vi "Rx Core 2945 2955.vi"(0 "rx.ddc parameters":T1[](array[typedef]) {"frequency shift" format="%#.48g"}, 1 "rx.samples to acquire":u32, 2 "Simulate Data":bool, 3 "rx.abort":bool, 4 "rx.stream enable":bool[](array[boolean]), 5 "rx.start trigger":bool, 6 "rx.reset":bool=TRUE, 7 "fifo 2":refnum<k21>, 10 "fifo 0":refnum<k21>, 11 "fifo 3":refnum<k21>, 12 "fifo 1":refnum<k21>) -> (13 "rx.dsp reset done":bool, 14 "rx.state":T3, 15 "rx.samples processed":u32, 17 "rx.number of fifo overflows":u32, 18 "rx.number of iq data overflows":u64[](array[numeric]))   [LabVIEW 2016]
uses:
  Stream Control State.ctl
  DDC Parameters.ctl
  <instrlib>/_niInstr/DSP/v1/Shared/Public/IQ Impairments.ctl
  <vilib>/rvi/eio/common/nirviEmuTemplateMethod_errors.vi
  <instrlib>/_niInstr/DSP/v1/FPGA/Public/Sub VIs/Data Conversion/I16 to IQ - 1 spc - S18.1.vi
  <instrlib>/_niInstr/Basic Elements/v1/FPGA/Private/Count Up U32.vi
  <vilib>/eio/EIONode/EIONode.xnode
  <instrlib>/_niInstr/Basic Elements/v1/FPGA/niInstr Basic Elements v1 FPGA.lvlib
  <instrlib>/_niInstr/DSP/v1/FPGA/niInstr DSP v1 FPGA.lvlib
  <instrlib>/_niInstr/DSP/v1/Shared/niInstr DSP v1 Shared.lvlib
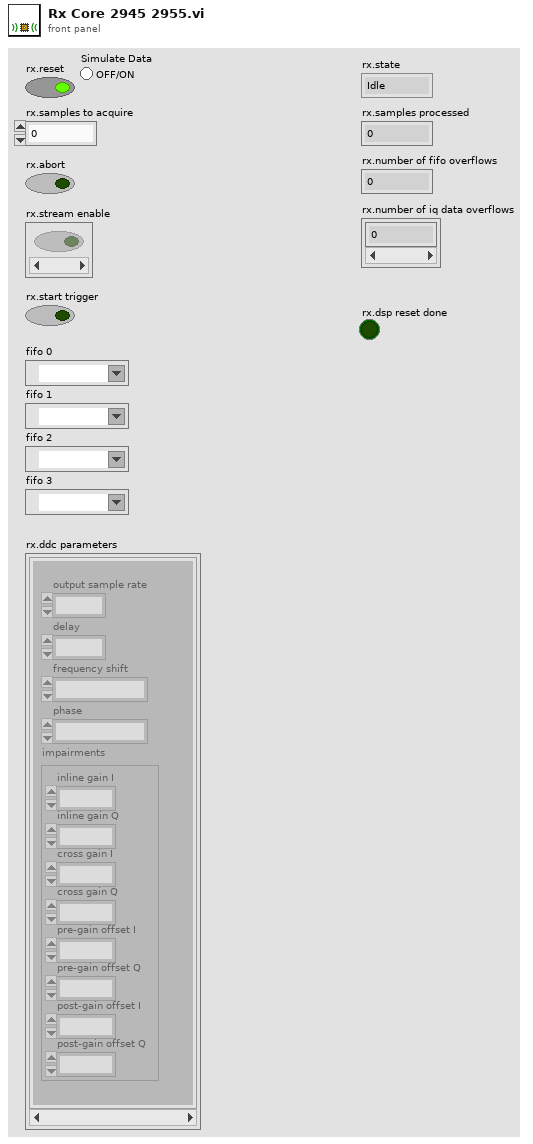
[diagram p1: front panel]
types:
  T1 = typedef "DDC Parameters.ctl" = cluster{"output sample rate":fxp<+,48,1>, "delay":fxp<+/-,16,0>, "frequency shift":fxp<+/-,48,0>, "impairments":T2, "phase":fxp<+/-,21,0>}
  T2 = typedef "niInstr DSP v1 Shared.lvlib/IQ Impairments.ctl" = cluster{"inline gain I":fxp<+/-,18,1>, "inline gain Q":fxp<+/-,18,1>, "cross gain I":fxp<+/-,18,1>, "cross gain Q":fxp<+/-,18,1>, "pre-gain offset I":fxp<+/-,18,1>, "pre-gain offset Q":fxp<+/-,18,1>, "post-gain offset I":fxp<+/-,18,1>, "post-gain offset Q":fxp<+/-,18,1>}
  T3 = typedef "Stream Control State.ctl" = enum16{"Idle", "Active"}
  T4 = typedef "niInstr DSP v1 Shared.lvlib/IQ Data.ctl" = cluster{"I":fxp<+/-,18,1>, "Q":fxp<+/-,18,1>, "overflow":bool}
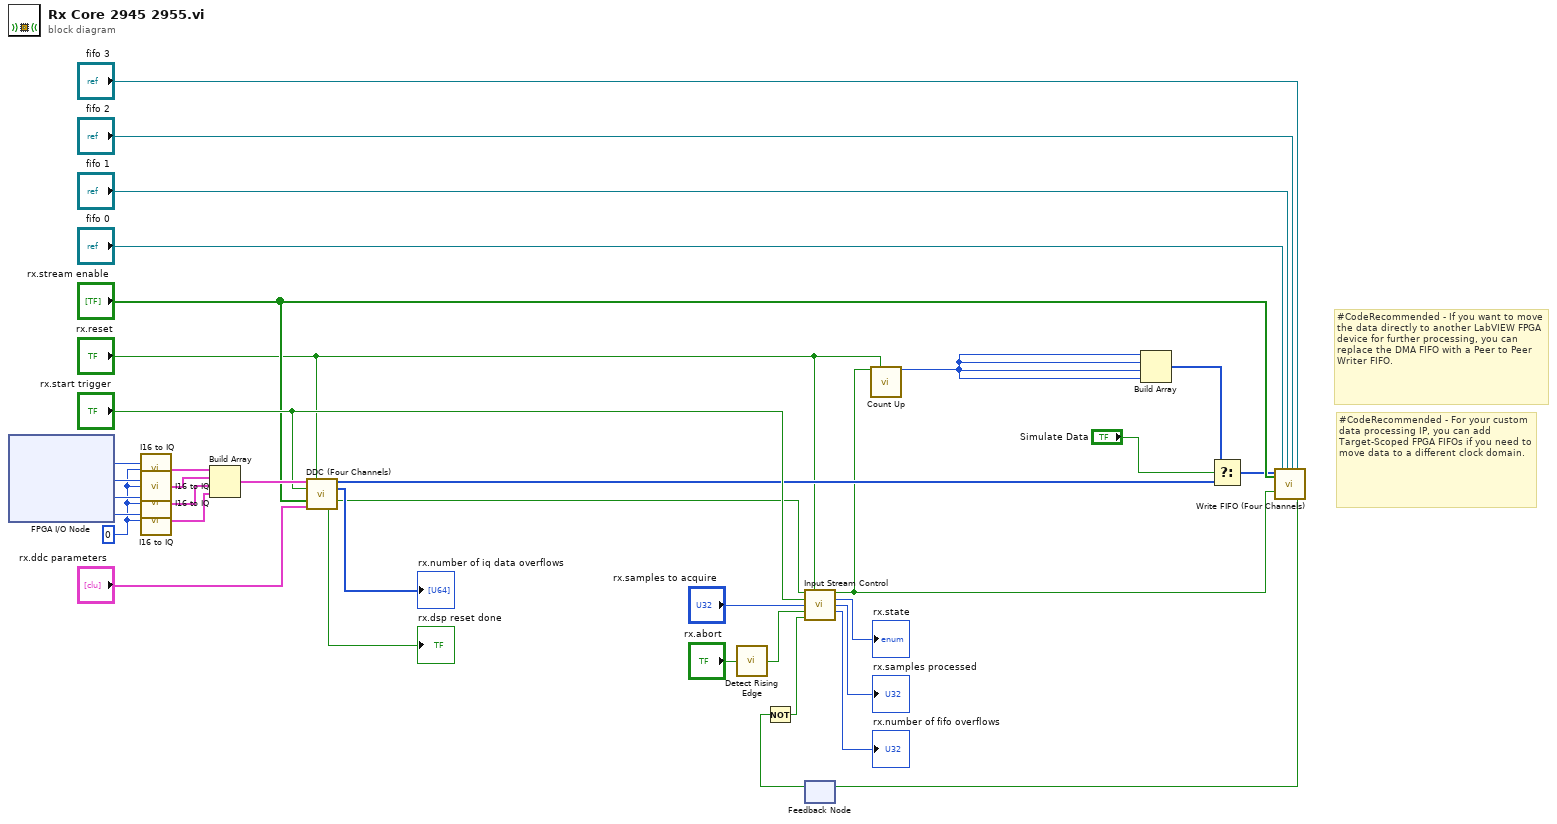
[diagram p0: block diagram]
diagram:
  w22 = i16 0 ("Q")
  # "#CodeRecommended - For your custom data processing IP, you can add Target-Scoped FPGA FIFOs if you need to move data to a different clock domain."
  # "#CodeRecommended - If you want to move the data directly to another LabVIEW FPGA device for further processing, you can replace the DMA FIFO with a Peer to Peer Writer FIFO."
  n1 = xnode "FPGA I/O Node"() -> ("RF 0/Rx/Rx1"=w26:i16, "RF 0/Rx/Rx2"=w25:i16, "RF 1/Rx/Rx1"=w24:i16, "RF 1/Rx/Rx2"=w23:i16)  [unwired: 4 in, 4 out]
  n2 = call-poly <instrlib>:"I16 to IQ.vi"("I"=w26, "Q"=w22) -> ("IQ"=w35:T4)  [unwired: 13 in]
  n3 = call-poly <instrlib>:"I16 to IQ.vi"("I"=w25, "Q"=w22) -> ("IQ"=w36:T4)  [unwired: 13 in]
  n4 = call-poly <instrlib>:"I16 to IQ.vi"("I"=w24, "Q"=w22) -> ("IQ"=w20:T4)  [unwired: 13 in]
  n5 = call-poly <instrlib>:"I16 to IQ.vi"("I"=w23, "Q"=w22) -> ("IQ"=w21:T4)  [unwired: 13 in]
  n6 = Build Array(w35, w36, w20, w21) -> (w14:T4[])
  n7 = call "DDC (Four Channels).vi"("data in"=w14, "reset"="rx.reset", "start trigger"="rx.start trigger", "enable"="rx.stream enable", "ddc parameters"="rx.ddc parameters") -> ("data out"=w7:u32[], "number of overflows"=→"rx.number of iq data overflows":u64[], "output valid"=w10:bool, "dsp reset done"=→"rx.dsp reset done":bool)  [unwired: 7 in]
  n8 = call <instrlib>:"Detect Rising Edge.vi"("signal"="rx.abort") -> ("edge detected"=w34:bool)  [unwired: 14 in]
  n9 = feedback #1() -> (w27:bool)  [unwired: 1 in]
  n10 = Not(x=w27) -> (.not. x?=w31:bool)
  n11 = call "Input Stream Control.vi"("input valid"=w10, "reset"="rx.reset", "start trigger"="rx.start trigger", "burst size"="rx.samples to acquire", "abort"=w34, "fifo timeout"=w31) -> ("write stream"=w3:bool, "state"=→"rx.state":T3, "samples processed"=→"rx.samples processed":u32, "number of overflows"=→"rx.number of fifo overflows":u32)  [unwired: 5 in, 1 out]
  n12 = call-poly <instrlib>:"Count Up.vi"("increment"=w3, "reset"="rx.reset") -> ("count out"=w1:u32)  [unwired: 13 in]
  n13 = Build Array(w1, w1, w1, w1) -> (w6:u32[])
  n14 = Select(t=w6, s="Simulate Data", f=w7) -> (s? t:f=w5:u32[])
  n15 = call "Write FIFO (Four Channels).vi"("data in"=w5, "enable"="rx.stream enable", "input valid"=w3, "fifo 0"="fifo 0", "fifo 1"="fifo 1", "fifo 2"="fifo 2", "fifo 3"="fifo 3") -> ("ready for input"=w17:bool)  [unwired: 12 in]
  n16 = feedback-in #1(w17) -> ()
